vi "readPre.vi"(1 "size":i32, 2 "address":u8, 3 "Channel":u8 max=5 step=1, 4 "input_order":u8[](array[numeric])=[238, 0, 13, 0, 0, 160, 0, 0, 169, 255, 252, 255, 255] format="%.0x") -> (0 "out":u8[](array[numeric]))   [LabVIEW 2011]
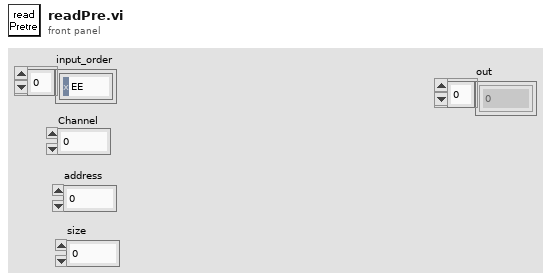
[diagram p1: front panel]
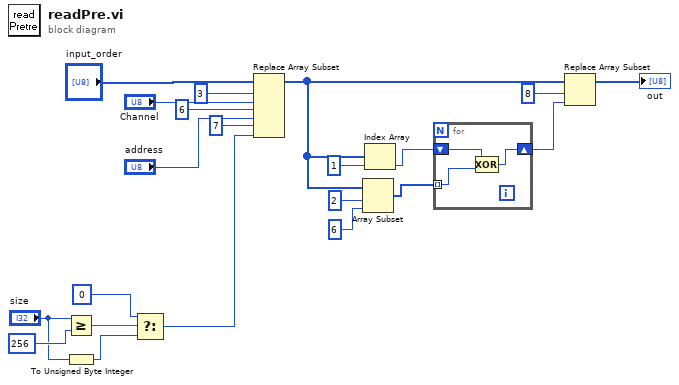
[diagram p0: block diagram]
diagram:
  n1 = Greater Or Equal?(x="size", y=256) -> (x >= y?=w6:bool)
  n2 = To Unsigned Byte Integer(number="size") -> (unsigned 8bit integer=w4:u8)
  n3 = Select(t=u8 0, s=w6, f=w4) -> (s? t:f=w2:u8)
  n4 = Replace Array Subset(array="input_order", new element #1="Channel", index #1=3 ("索引"), new element #2="address", index #2=6 ("索引"), new element #3=w2, index #3=7 ("索引")) -> (w11:u8[])
  n5 = Array Subset(array=w11, index=2 ("索引"), length=6 ("长度")) -> (w12:u8[])
  n6 = Index Array(array=w11, index=1 ("索引")) -> (element=w13:u8)
  n7 = for {
    shift-right: [w22] -> w9
    shift-left: w13 -> [w24]
    tunnel: w12 -> [w23] mode=indexing
    n8 = Compound Arithmetic op=XOR(w24, w23) -> (w22:u8)
  }
  n9 = Replace Array Subset(array=w11, new element=w9, index=8 ("索引")) -> (→"out":u8[])
